vi "Set Value.vi"(8 "error in (no error)":errorcluster, 10 "Variant":variant, 11 "Refnum Value Source in":refnum<class "Ctrl Refnum Value Source.lvclass">) -> (0 "error out":errorcluster, 3 "Refnum Value Source out":refnum<class "Ctrl Refnum Value Source.lvclass">)   [LabVIEW 2020, in "Composed Columns.lvlib" / "Ctrl Refnum Value Source.lvclass"]
uses:
  Ctrl Refnum Value Source.lvclass
  Ctrl Refnum Value Source.lvclass/Ctrl Refnum Value Source.ctl
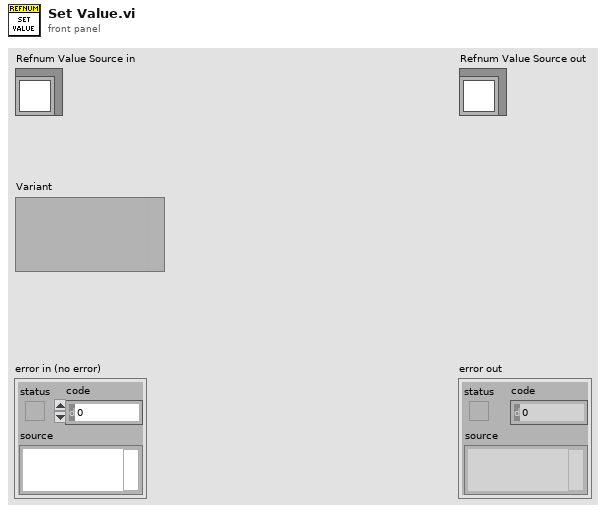
[diagram p1: front panel]
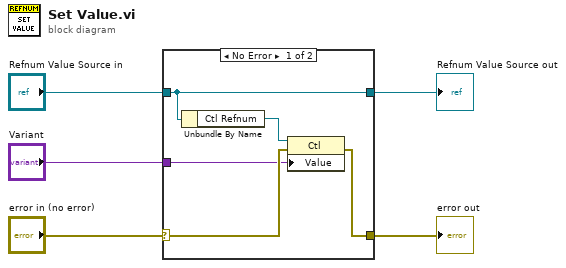
[diagram p0: block diagram]
diagram:
  n1 = case shown="No Error" "error in (no error)" {
    selector: "error in (no error)" -> [w8 w12]
    tunnel: [w6 w12] -> w4
    tunnel: "Refnum Value Source in" -> [w10 w11]
    tunnel: [w10 w11] -> w2
    tunnel: "Variant" -> [w7 _]
    frame No Error {
      n2 = Unbundle By Name(w10) -> ("Ctl Refnum"=w9:refnum<vi>)
      n3 = property class="Ctl"(reference=w9, error in=w8, "Value"=w7) -> (error out=w6:errorcluster)  [unwired: 1 out]
    }
    frame Error {
    }
  }
  "error out" <- w4
  "Refnum Value Source out" <- w2
